vi "Serial_Init.vi"(3 "error in (no error)":errorcluster) -> (0 "error out":errorcluster, 2 "Serial Ref":T1)   [LabVIEW 2009, in "Serial.lvlib"]
doc: "Initializes serial port on compact RIO. Creates a semaphore for data sending. Sets the VISA Ref variable.\nThis VI must be executed prior to any other VI that uses serial port."
uses:
  Serial.lvlib
  Serial Ref.ctl
  <vilib>/Instr/_visa.llb/VISA Configure Serial Port (Instr).vi
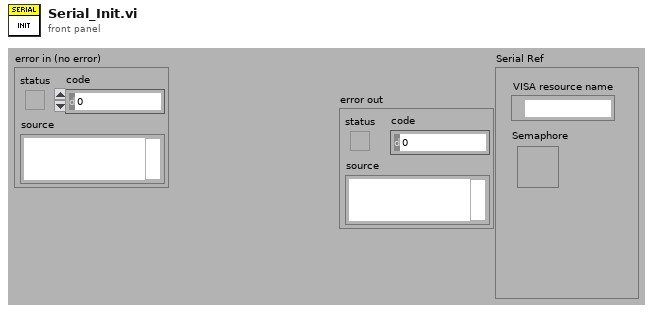
[diagram p1: front panel]
types:
  T1 = typedef "Serial.lvlib/Serial Ref.ctl" = cluster{"VISA resource name":refnum<visa-resource-name>, "Semaphore":T2}
  T2 = typedef "Semaphore RefNum" = refnum<k1>
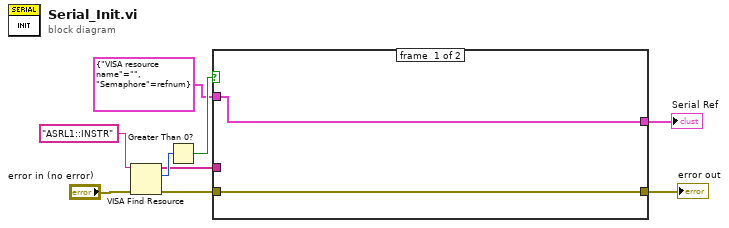
[diagram p0: block diagram]
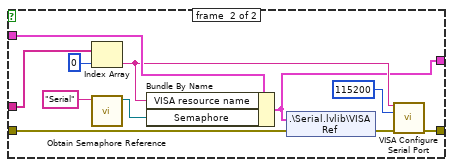
[diagram p2: hidden frame]
diagram:
  n1 = VISA Find Resource(8:"error in (no error)", 11:"ASRL1::INSTR" ("expression (\"?*\")")) -> (0:w4:errorcluster, 2:w8:u32, 3:w6:string[])  [unwired: 1 in]
  n2 = Greater Than 0?(x=w8) -> (x > 0?=w7:bool)
  n3 = case shown="True" w7 {
    tunnel: w6 -> [_ w22]
    tunnel: w4 -> [w11 w18]
    tunnel: [w10 w12] -> w1
    tunnel: [w11 w20] -> w3
    tunnel: T1 {"VISA resource name"="", "Semaphore"=refnum} ("Serial Ref") -> [w10 w15]
    frame #0 {
    }
    frame #1 {
      n4 = Index Array(array=w22, index=0) -> (element=w14:string)
      n5 = call <vilib>:"Obtain Semaphore Reference.vi"("name (unnamed)"="Serial") -> ("semaphore"=w13:T2)  [unwired: 4 in, 2 out]
      n6 = Bundle By Name(cluster=w15, "VISA resource name"=w14, "Semaphore"=w13) -> (w12:T1)
      n7 = shared-variable ".\\Serial.lvlib\\VISA Ref"(w12, error in=w18) -> (error out=w17:errorcluster)
      n8 = call-poly "VISA Configure Serial Port"("VISA resource name"=w14, "baud rate (9600)"=u32 115200, "error in (no error)"=w17) -> ("error out"=w20:errorcluster)  [unwired: 11 in, 1 out]
    }
  }
  "error out" <- w3
  "Serial Ref" <- w1
